vi "DSF.Engine.Framework.Get Plugins.vi"(11 "Framework in":refnum<class "DSF.Engine.Framework.lvclass">) -> (2 "Plugins":refnum<class "DSF.Engine.Plugin.lvclass">[](array[class]), 3 "Framework out":refnum<class "DSF.Engine.Framework.lvclass">)   [LabVIEW 2017, in "DSF.Engine.lvlib" / "DSF.Engine.Framework.lvclass"]
uses:
  DSF.Engine.Framework.lvclass
  Plugin/DSF.Engine.Plugin.lvclass
  DSF.Engine.Framework.lvclass/DSF.Engine.Framework.ctl
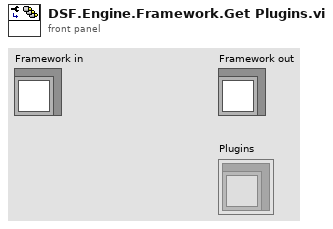
[diagram p1: front panel]
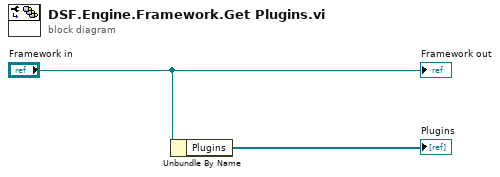
[diagram p0: block diagram]
diagram:
  n1 = Unbundle By Name("Framework in") -> ("Plugins"=→"Plugins":refnum<class "DSF.Engine.Plugin.lvclass">[])
  "Framework out" <- "Framework in"
